vi "多参数校准写入.vi"(8 "Error in":errorcluster caption="Error in (no error)", 9 "B":dbl caption="校准值B:", 10 "K":dbl caption="校准值K:", 11 "站号":u16(ring)=10 items=["氨氮"=3, "水温"=9, "pH值"=10, "电导率"=12, "浊度"=13, "叶绿素a"=14, "藻密度"=15, "蓝绿藻"=16, "氧化还原电位"=17, "溶解氧%"=18, "盐度"=19]) -> (0 "error out":errorcluster)   [LabVIEW 2016, in "斯坦道仪器.lvlib"]
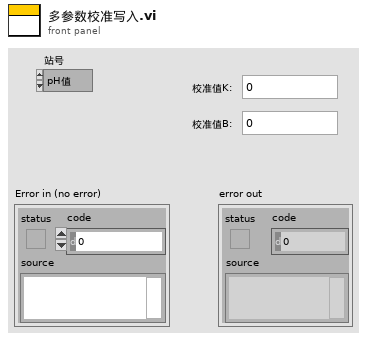
[diagram p1: front panel]
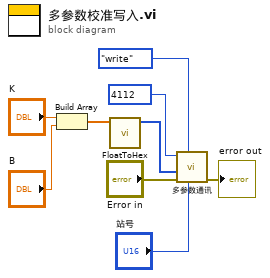
[diagram p0: block diagram]
diagram:
  n1 = Build Array("K", "B") -> (w3:dbl[])
  n2 = call "FloatToHex.vi"("浮点数"=w3) -> ("DCBA整形输出"=w2:u16[])  [unwired: 10 in]
  n3 = call "多参数通讯.vi"("Slave ID"="站号", "STEP"=enum16{"open", "read", "write", "close"}."write", "Error in"="Error in", "values"=w2, "starting address"=u16 4112) -> ("error out"=→"error out":errorcluster)  [unwired: 4 in, 2 out]
